vi "PolinomEğri.vi"() -> ()   [LabVIEW 2015]
uses:
  <vilib>/Utility/file.llb/Read Delimited Spreadsheet (DBL).vi
  <vilib>/Analysis/NI_AALPro.lvlib
panel:
  in  "Polinom Derecesi":dbl
  out "POLİNOM EĞRİ UYDURMA":dbl[](graph)
  out "Veriler":dbl[][](array[numeric])
  in  "Okunacak Veri Adresi":path
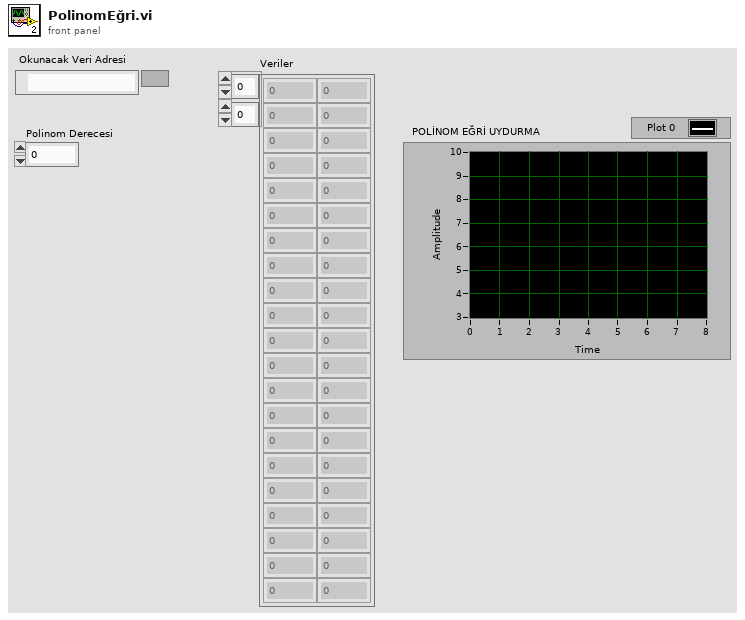
[diagram p1: front panel]
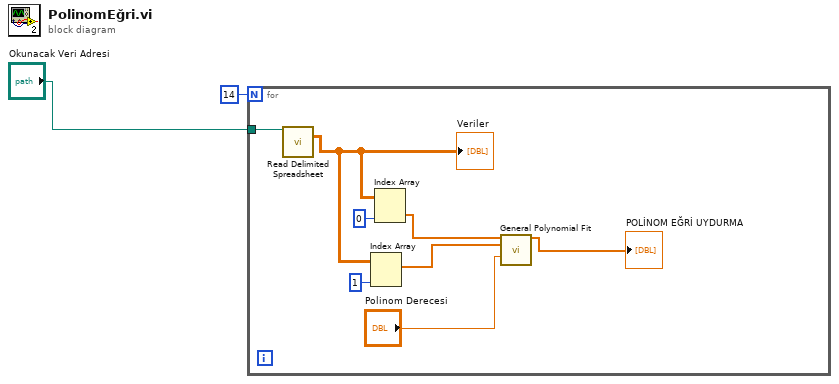
[diagram p0: block diagram]
diagram:
  n1 = for {
    N: 14 -> [_]
    tunnel: "Okunacak Veri Adresi" -> [w10]
    n2 = call-poly <vilib>:"Read Delimited Spreadsheet.vi"("file path (dialog if empty)"=w10) -> ("all rows"=w8:dbl[][])  [unwired: 9 in, 5 out]
    "Veriler" <- w8
    n3 = Index Array(array=w8, index (col)=1 ("disabled index (col)")) -> (element=w5:dbl[])  [unwired: 1 in]
    n4 = Index Array(array=w8, index (col)=0 ("disabled index (col)")) -> (element=w6:dbl[])  [unwired: 1 in]
    n5 = call <vilib>:"General Polynomial Fit.vi"("Y"=w6, "X"=w5, "tolerance"="Polinom Derecesi") -> ("Best Polynomial Fit"=→"POLİNOM EĞRİ UYDURMA":dbl[])  [unwired: 9 in, 3 out]
  }
